vi "sub_SignalProcessing.vi"(7 "nulling":bool, 8 "error in":errorcluster, 11 "Q_data":T2) -> (0 "error out":errorcluster, 3 "log data":T1)   [LabVIEW 2016]
uses:
  ctl/q_data.ctl
  ctl/log_data.ctl
  ctl/Data_buf_cmd.ctl
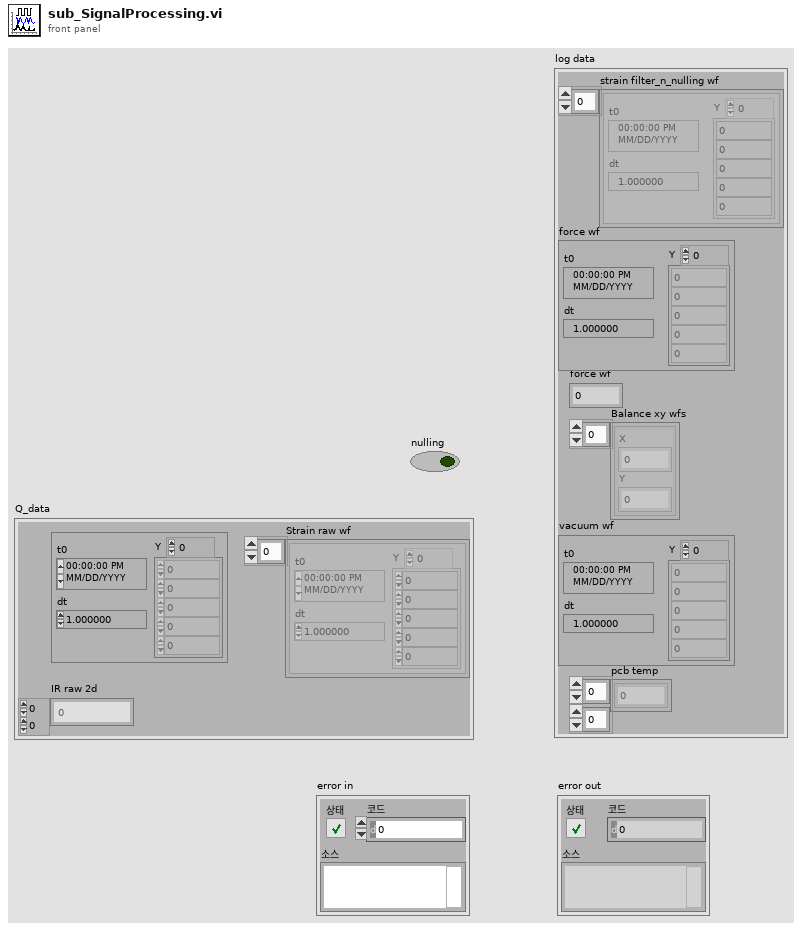
[diagram p1: front panel]
types:
  T1 = typedef "log_data.ctl" = cluster{"strain filter_n_nulling wf":waveform(dbl)[], "force wf":waveform(dbl), "force":dbl, "Balance xy wfs":cluster{"X":dbl, "Y":dbl}[], "vacuum kpa wf":waveform(dbl), "pcb temp":dbl[][]}
  T2 = typedef "q_data.ctl" = cluster{"Strain raw wf":waveform(dbl)[], "vacuum raw wf":waveform(dbl), "IR raw 2d":i16[][]}
  T3 = typedef "Data_buf_cmd.ctl" = enum16{"insert", "default", "create", "clear"}
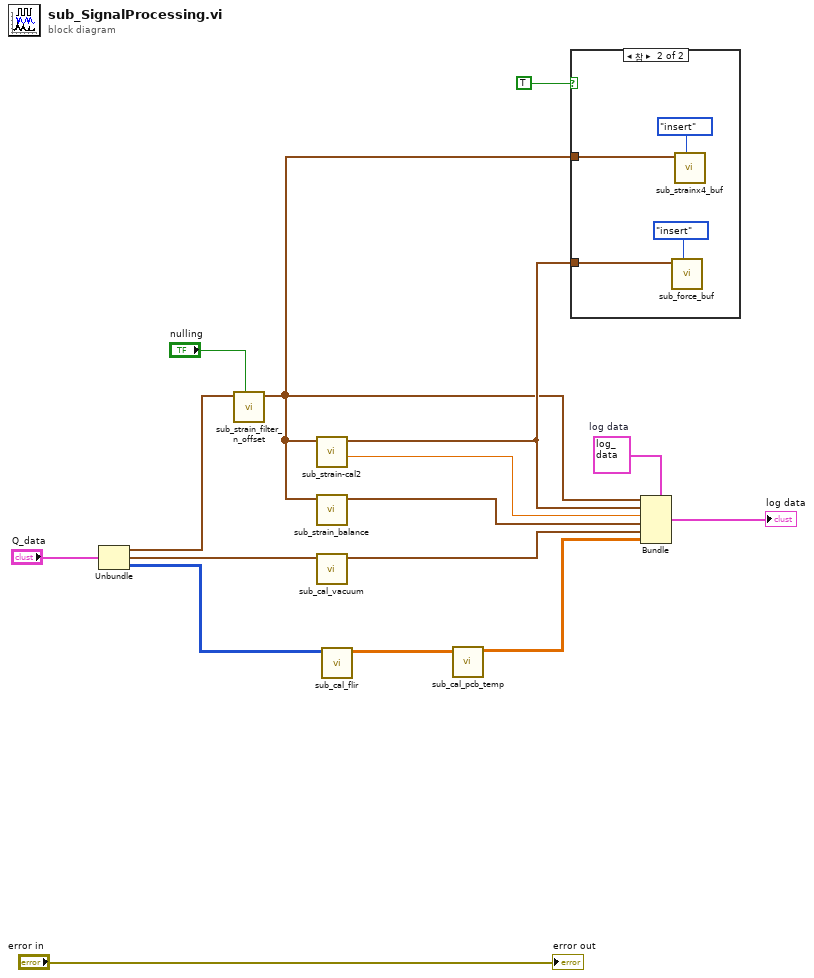
[diagram p0: block diagram]
diagram:
  w11 = T1 {"strain filter_n_nulling wf"=[], "force wf"={"t0"=timestamp(0 s since 1904-01-01), "dt"=1.0, "Y"=[]}, "force"=0.0, "Balance xy wfs"=[], "vacuum kpa wf"={"t0"=timestamp(0 s since 1904-01-01), "dt"=1.0, "Y"=[]}, "pcb temp"=[]}  # log data
  n1 = Unbundle("Q_data") -> ("Strain raw wf"=w9:waveform(dbl)[], "vacuum raw wf"=w8:waveform(dbl), "IR raw 2d"=w7:i16[][])
  n2 = call "sub_strain_filter_n_offset.vi"("nulling"="nulling", "Strain raw wf"=w9) -> ("strain filter_n_nulling wf"=w1:waveform(dbl)[])  [unwired: 9 in]
  n3 = call "sub_strain-cal2.vi"("strain wfs"=w1) -> ("force"=w13:dbl, "force wf"=w3:waveform(dbl))  [unwired: 9 in]
  n4 = call "sub_strain_balance.vi"("strain_offset_wf"=w1) -> ("Balance xy wfs"=w12:cluster{"X":dbl, "Y":dbl}[])  [unwired: 9 in, 1 out]
  n5 = call "sub_cal_vacuum.vi"("vacuum v wf"=w8) -> ("vacuum kpa wf"=w14:waveform(dbl))  [unwired: 10 in]
  n6 = call "sub_cal_flir.vi"("FLIR cam data"=w7) -> ("temp data"=w5:dbl[][])  [unwired: 10 in]
  n7 = call "sub_cal_pcb_temp.vi"("ir temp"=w5) -> ("pcb temp"=w16:dbl[][])  [unwired: 10 in]
  n8 = case shown="참" TRUE {
    tunnel: w3 -> [_ w19]
    tunnel: w1 -> [_ w17]
    frame False {
    }
    frame True {
      n9 = call "sub_force_buf.vi"("cmd"=Data_buf_cmd."insert", "forcewf"=w19) -> ()  [unwired: 8 in, 2 out]
      n10 = call "sub_strainx4_buf.vi"("cmd"=Data_buf_cmd."insert", "strain filter_n_nulling wf"=w17) -> ()  [unwired: 8 in, 2 out]
    }
  }
  n11 = Bundle(cluster=w11, "strain filter_n_nulling wf"=w1, "force wf"=w3, "force"=w13, "Balance xy wfs"=w12, "vacuum kpa wf"=w14, "pcb temp"=w16) -> (→"log data":T1)
  "error out" <- "error in"
